vi "读文件解析.vi"(9 "读取的字节":i32, 10 "响应":string) -> (1 "读文件":string[](array[string]), 2 "响应":bool)   [LabVIEW 2015]
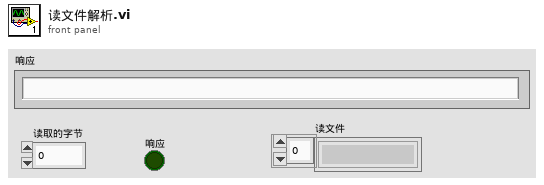
[diagram p1: front panel]
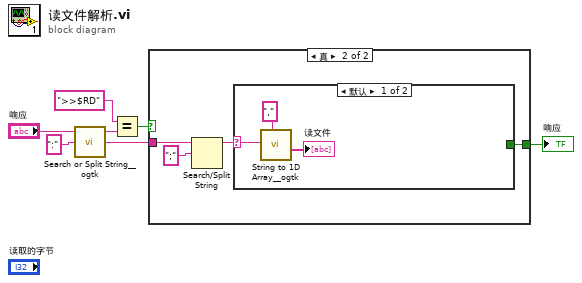
[diagram p0: block diagram]
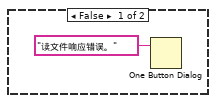
[diagram p2: hidden frame]
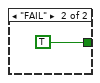
[diagram p3: hidden frame]
diagram:
  n1 = call <userlib>:"Search or Split String__ogtk.vi"("search string/char (-)"=":", "string"="响应") -> ("substring after match"=w2:string, "substring before match"=w5:string)  [unwired: 1 in, 1 out]
  n2 = Equal?(x=">>$RD" ("消息"), y=w5) -> (x = y?=w3:bool)
  n3 = case shown="真" w3 {
    tunnel: w2 -> [_ w11]
    tunnel: [_ w9] -> w1
    frame False {
      n4 = One Button Dialog(message="读文件响应错误。" ("消息")) -> ()  [unwired: 1 in, 1 out]
    }
    frame True {
      n5 = Search/Split String(string=w11, search string/char (-)=";" ("搜索字符串/字符(-)")) -> (substring before match=w10:string)  [unwired: 1 in, 2 out]
      n6 = case shown="默认" w10 {
        selector: w10 -> [w15 _]
        tunnel: [_ TRUE] -> w9
        frame Default {
          n7 = call <userlib>:"String to 1D Array__ogtk.vi"("delimiter (Tab)"=",", "string"=w15) -> ("Array of Strings"=→"读文件":string[])  [unwired: 9 in]
        }
        frame "FAIL" {
        }
      }
    }
  }
  "响应" <- w1
